vi "text파일로 저장되어 있는 위도경도 데이터 k, k+1, k+2점 분리 & 거리, 방향각, 조향각 계산.vi"() -> ()   [LabVIEW 2016]
uses:
  DLL/bearingP1toP2.dll
  DLL/distance_of_P1toP2.dll
panel:
  out "Latitude 1":string
  out "Longitude 1":string
  out "Latitude 2":string
  out "Longitude 2":string
  out "Bearing angle 1 (deg)":u16
  out "Distance (m)":dbl format="%#.6g"
  out "k번째":i32
  out "(k+1)번째":i32
  out "Latitude 3":string
  out "Longitude 3":string
  out "(k+2)번째":i32
  out "Steering angle (deg)":i16
  in  "파일(대화 상자 사용)":path=path "C:/Users/user/Desktop/작업중인 모든 Vi, dll파일 모음/Global Mapping Data.txt"
  in  "?":i32=1
  out "Bearing angle 2 (deg)":u16
  # "번째 경유점"
  # "번째 경유점"
  # "번째 경유점"
  # "k번째 경유점"
  # "Bearing\n angle"
  # "Steering\n  angle"
  # "Distance"
  # "m"
  # "deg"
  # "deg"
  # "="
  # "="
  # "="
  # "k  ="
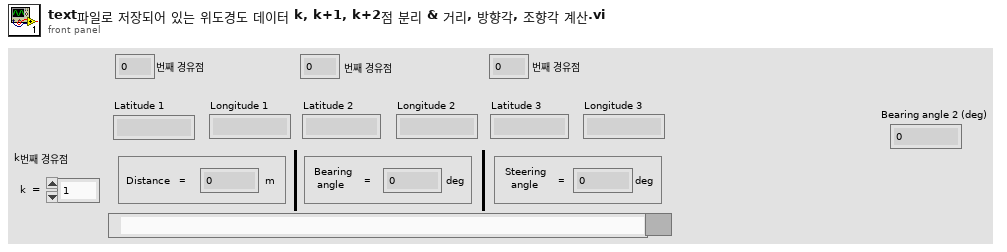
[diagram p1: front panel]
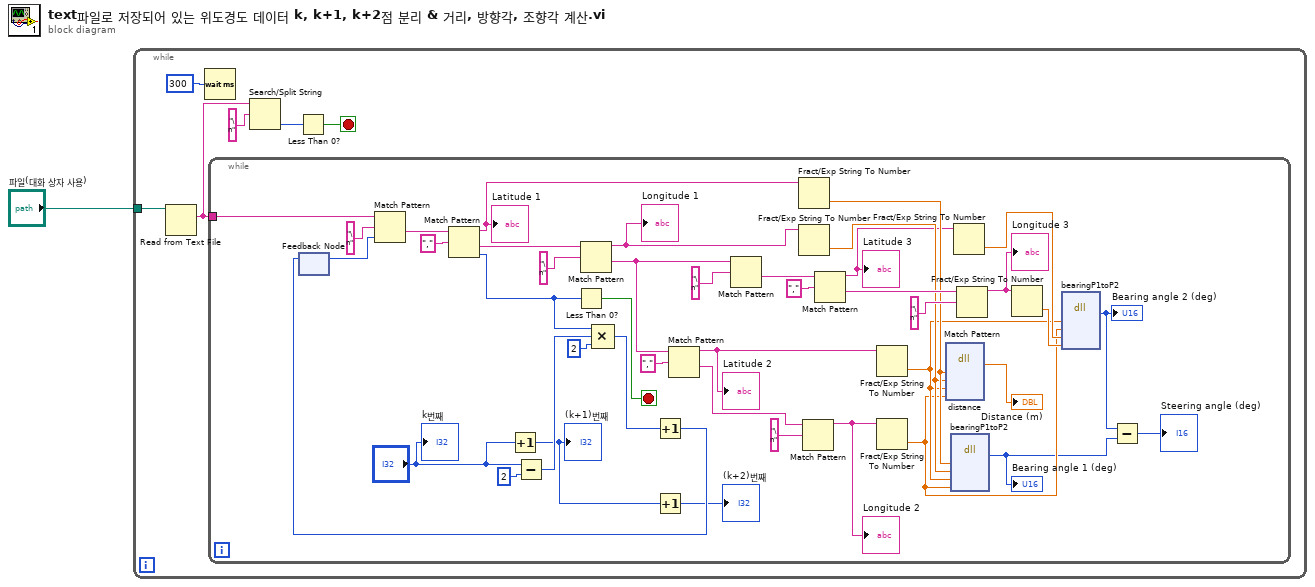
[diagram p0: block diagram]
diagram:
  n1 = while {
    tunnel: "파일(대화 상자 사용)" -> [w3]
    stop <- w6 stop-if-true
    n2 = Read from Text File(file (use dialog)=w3) -> (text=w2:string)  [unwired: 3 in, 3 out]
    n3 = Wait (ms)(milliseconds to wait=u32 300 ("대기 시간 (ms)")) -> ()  [unwired: 1 out]
    n4 = while {
      tunnel: w2 -> [w44]
      stop <- w49 stop-if-true
      n5 = feedback #1() -> (w35:i32)  [unwired: 1 in]
      n6 = Match Pattern(string=w44, regular expression="\n" ("정규식"), offset (0)=w35) -> (after substring=w43:string)  [unwired: 3 out]
      n7 = Match Pattern(string=w43, regular expression="," ("search string/char (-)")) -> (before substring=w34:string, after substring=w47:string, offset past match=w38:i32)  [unwired: 1 in, 1 out]
      "Latitude 1" <- w34
      n8 = Increment(x="?") -> (x+1=w19:i32)
      "(k+1)번째" <- w19
      n9 = Subtract(x="?", y=2) -> (x-y=w28:i32)
      n10 = Less Than 0?(x=w38) -> (x < 0?=w49:bool)
      n11 = Match Pattern(string=w47, regular expression="\n" ("정규식")) -> (before substring=w33:string, after substring=w26:string)  [unwired: 1 in, 2 out]
      "Longitude 1" <- w33
      n12 = Compound Arithmetic op=MULTIPLY(w38, w28, 2 ("값")) -> (w37:i32)
      n13 = Increment(x=w37) -> (x+1=w36:i32)
      n14 = feedback-in #1(w36) -> ()
      n15 = Increment(x=w19) -> (x+1=→"(k+2)번째":i32)
      n16 = Match Pattern(string=w26, regular expression="," ("search string/char (-)")) -> (before substring=w32:string, after substring=w40:string)  [unwired: 1 in, 2 out]
      "Latitude 2" <- w32
      n17 = Match Pattern(string=w26, regular expression="\n" ("정규식")) -> (after substring=w24:string)  [unwired: 1 in, 3 out]
      n18 = Fract/Exp String To Number(string=w34) -> (number=w18:dbl)  [unwired: 3 in, 1 out]
      n19 = Fract/Exp String To Number(string=w33) -> (number=w17:dbl)  [unwired: 3 in, 1 out]
      n20 = Match Pattern(string=w40, regular expression="\n" ("정규식")) -> (before substring=w31:string)  [unwired: 1 in, 3 out]
      "Longitude 2" <- w31
      n21 = Match Pattern(string=w24, regular expression="," ("정규식")) -> (before substring=w16:string, after substring=w22:string)  [unwired: 1 in, 2 out]
      "Latitude 3" <- w16
      n22 = Fract/Exp String To Number(string=w32) -> (number=w12:dbl)  [unwired: 3 in, 1 out]
      n23 = Fract/Exp String To Number(string=w31) -> (number=w11:dbl)  [unwired: 3 in, 1 out]
      n24 = dll-call lib="PTH2abs CUsersuserDesktop[Github]_GPS Teamlabview_program(ììì¤ì¸ ëª¨ë  Vi, dllíì¼ ëª¨ìì ì²´íë¡ê·¸ë¨DLLdistance_of_P1toP2.dll" fn="distance" label="사이 거리"("P1_latitude"=w18, "P1_longitude"=w17, "P2_latitude"=w12, "P2_longitude"=w11) -> ("반환 타입"=→"Distance (m)":dbl)  [unwired: 7 in, 2 out]
      n25 = dll-call lib="PTH2abs CUsersuserDesktop[Github]_GPS Teamlabview_program(ììì¤ì¸ ëª¨ë  Vi, dllíì¼ ëª¨ìì ì²´íë¡ê·¸ë¨DLLbearingP1toP2.dll" fn="bearingP1toP2" label="방향각"("P1_latitude"=w18, "P1_longitude"=w17, "P2_latitude"=w12, "P2_longitude"=w11) -> ("반환 타입"=w9:u16)  [unwired: 7 in, 2 out]
      "Bearing angle 1 (deg)" <- w9
      n26 = Fract/Exp String To Number(string=w16) -> (number=w15:dbl)  [unwired: 3 in, 1 out]
      n27 = Match Pattern(string=w22, regular expression="\n" ("정규식")) -> (before substring=w14:string)  [unwired: 1 in, 3 out]
      "Longitude 3" <- w14
      n28 = Fract/Exp String To Number(string=w14) -> (number=w13:dbl)  [unwired: 3 in, 1 out]
      n29 = dll-call lib="PTH2abs CUsersuserDesktop[Github]_GPS Teamlabview_program(ììì¤ì¸ ëª¨ë  Vi, dllíì¼ ëª¨ìì ì²´íë¡ê·¸ë¨DLLbearingP1toP2.dll" fn="bearingP1toP2" label="방향각"("P1_latitude"=w12, "P1_longitude"=w11, "P2_latitude"=w15, "P2_longitude"=w13) -> ("반환 타입"=w10:u16)  [unwired: 7 in, 2 out]
      "Bearing angle 2 (deg)" <- w10
      n30 = Subtract(x=w10, y=w9) -> (x-y=→"Steering angle (deg)":u16)
      "k번째" <- "?"
    }
    n31 = Search/Split String(string=w2, search string/char (-)="\n") -> (offset of match=w5:i32)  [unwired: 3 out]
    n32 = Less Than 0?(x=w5) -> (x < 0?=w6:bool)
  }
